vi "PH_PSDBWriter.PC get Shot ID.vi"(0 "i ref in":refnum<vi>, 2 "Data":T1, 5 "error IO":errorcluster) -> (14 "i ref in":refnum<vi>, 19 "error IO":errorcluster)   [LabVIEW 2014, in "PH_PSDBWriter.lvlib"]
doc: "This VI gets the curent shot number and sets it to own attributes."
uses:
  PH_PSDBWriter.lvlib
  CSCore/CSSystem/CoreDefs/CoreDefs.rawDataType.ctl
  CSCore/CAEObj/CAEObj.lvlib
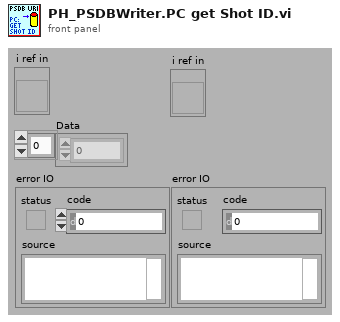
[diagram p1: front panel]
types:
  T1 = typedef "CoreDefs.rawDataType.ctl" = i8[]
  T2 = typedef "PH_PSDBWriter.lvlib/PH_PSDBWriter.i attribute.ctl" = cluster{"PSDB Status Service ID":i32, "Instance ID":i32, "Shot #":i32, "Subsystem":T3, "Data Status":T4, "Ref PSDB Status":refnum<vi>, "PSDB Error Code":i32, "PSDB Dataset":T5, "PSDB Thread":cluster{"Ref":refnum<vi>, "Q-Ref":refnum<queue>}, "PSDB Credentials":T13}
  T3 = typedef "PH_PSDBWriter.lvlib/PH_PSDBWriter.PHELIX-Subsystems.ctl" = i32
  T4 = typedef "PH_PSDBWriter.lvlib/PH_PSDBWriter.Data Status.ctl" = i16
  T5 = typedef "PH_PSDBWriter.lvlib/PH_PSDBWriter.PSDB Dataset.ctl" = cluster{"Version":i32, "2D data Input":T6[], "Boolean Input":T8[], "Image Input":T9[], "Numeric Input":T11[], "String Input":T12[]}
  T6 = typedef "PH_PSDBWriter.lvlib/PH_PSDBWriter.2D dataset.ctl" = cluster{"name":string, "data":dbl[][], "axis description":T7}
  T7 = typedef "PSDB.lvlib/PSDB_AxisDescription.ctl" = cluster{"x axis label":string, "y axis label":string, "x axis unit":string, "y axis unit":string}
  T8 = typedef "PH_PSDBWriter.lvlib/PH_PSDBWriter.Boolean dataset.ctl" = cluster{"name":string, "data":bool, "unit":string}
  T9 = typedef "PH_PSDBWriter.lvlib/PH_PSDBWriter.Image dataset.ctl" = cluster{"name":string, "data":T10, "unit":string}
  T10 = typedef "IMAQ Image.ctl" = refnum<image>
  T11 = typedef "PH_PSDBWriter.lvlib/PH_PSDBWriter.Numeric dataset.ctl" = cluster{"name":string, "data":dbl, "unit":string}
  T12 = typedef "PH_PSDBWriter.lvlib/PH_PSDBWriter.String dataset.ctl" = cluster{"name":string, "data":string, "unit":string}
  T13 = typedef "PH_Common.lvlib/PH_Connection.PSDB Credentials.ctl" = cluster{"PW":string, "ID":string, "DS":string}
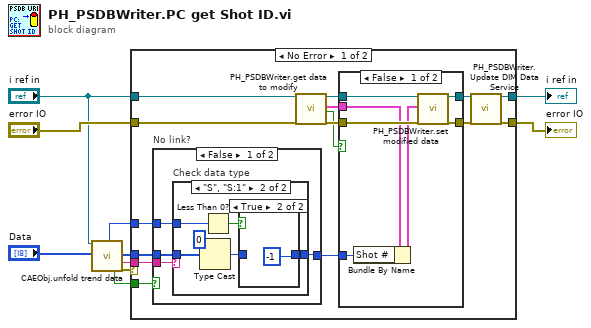
[diagram p0: block diagram]
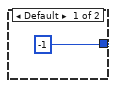
[diagram p3: hidden frame]
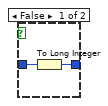
[diagram p4: hidden frame]
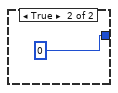
[diagram p5: hidden frame]
diagram:
  n1 = call "CAEObj.unfold trend data.vi"("i ref in"="i ref in", "raw trend data"="Data") -> ("quality"=w1:i32, "no link"=w5:bool, "data"=w2:i8[], "typeDescriptor"=w3:string, "error out"=w4:errorcluster)  [unwired: 9 in, 4 out]
  n2 = case shown="No Error" w4 {
    tunnel: "error IO" -> [w21 w51]
    tunnel: [w14 w50] -> w7
    tunnel: [w12 w51] -> w9
    tunnel: "i ref in" -> [w20 w50]
    tunnel: w5 -> [w25 _]
    tunnel: w3 -> [w24 _]
    tunnel: w2 -> [w23 _]
    tunnel: w1 -> [w22 _]
    frame No Error {
      n3 = case "No link?" shown="False" w25 {
        tunnel: [w38 0] -> w15
        tunnel: w22 -> [w37 _]
        tunnel: w23 -> [w36 _]
        tunnel: w24 -> [w35 _]
        frame False {
          n4 = case "Check data type" shown="\"S\", \"S:1\"" w35 {
            tunnel: [-1 w45] -> w38
            tunnel: w37 -> [_ w43]
            tunnel: w36 -> [_ w41]
            frame Default {
            }
            frame "S", "S:1" {
              n5 = Type Cast(type=i16 0, x=w41) -> (*(type *) &x=w40:i16)
              n6 = Less Than 0?(x=w43) -> (x < 0?=w44:bool)
              n7 = case shown="True" w44 {
                tunnel: [w46 -1] -> w45
                tunnel: w40 -> [w47 _]
                frame False {
                  n8 = To Long Integer(number=w47) -> (32bit integer=w46:i32)
                }
                frame True {
                }
              }
            }
          }
        }
        frame True {
        }
      }
      n9 = call "PH_PSDBWriter.get data to modify.vi"("i ref in"=w20, "error in (no error)"=w21) -> ("i ref out"=w18:refnum<vi>, "i attribute"=w16:T2, "timed out"=w17:bool, "error out"=w19:errorcluster)  [unwired: 14 in]
      n10 = case shown="False" w17 {
        tunnel: w19 -> [w32 w33]
        tunnel: [w31 w33] -> w11
        tunnel: w18 -> [w30 w34]
        tunnel: [w29 w34] -> w13
        tunnel: w16 -> [w28 _]
        tunnel: w15 -> [w26 _]
        frame False {
          n11 = Bundle By Name(cluster=w28, "Shot #"=w26) -> (w27:T2)
          n12 = call "PH_PSDBWriter.set modified data.vi"("i ref in"=w30, "i attribute"=w27, "error in (no error)"=w32) -> ("i ref out"=w29:refnum<vi>, "error out"=w31:errorcluster)  [unwired: 15 in]
        }
        frame True {
        }
      }
      n13 = call "PH_PSDBWriter.Update DIM Data Service.vi"("i ref in"=w13, "error in"=w11) -> ("i ref out"=w14:refnum<vi>, "error out"=w12:errorcluster)  [unwired: 16 in]
    }
    frame Error {
    }
  }
  "error IO" <- w9
  "i ref in" <- w7
